vi "filterWheelOpen.vi"   [LabVIEW 2017]
uses:
  globalDevices.vi
  <vilib>/Instr/_visa.llb/VISA Configure Serial Port (Instr).vi
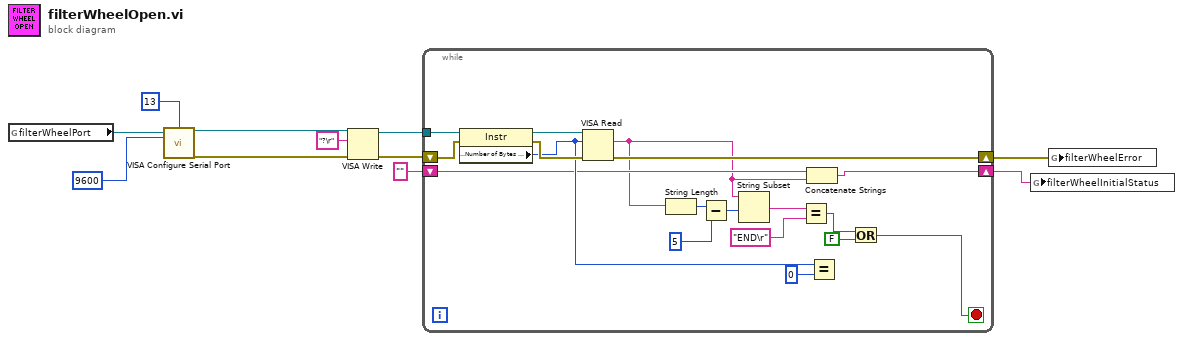
[diagram p0: block diagram]
diagram:
  n1 = global read "globalDevices.vi" "filterWheelPort"() -> (w10:refnum<visa-resource-name>)
  n2 = call-poly "VISA Configure Serial Port"("VISA resource name"=w10, "termination char\n(0xA = '\\n' = LF)"=u8 13 ("termination char\n(0xA = '\\n' = LF)"), "baud rate (9600)"=u32 9600) -> ("VISA resource name out"=w9:refnum<visa-resource-name>, "error out"=w8:errorcluster)  [unwired: 11 in]
  n3 = VISA Write(VISA resource name=w9, write buffer="?\r", error in (no error)=w8) -> (VISA resource name out=w6:refnum<visa-resource-name>, error out=w5:errorcluster)  [unwired: 1 out]
  n4 = while {
    tunnel: w6 -> [w29]
    shift-right: [w15] -> w2
    shift-left: "" -> [w16]
    shift-right: [w14] -> w3
    shift-left: w5 -> [w28]
    stop <- w17 stop-if-true
    n5 = property class="Instr"(reference=w29, error in=w28) -> (reference out=w27:refnum<visa-resource-name>, error out=w26:errorcluster, "Serial Settings:Number of Bytes at Serial Port"=w19:u32)
    n6 = VISA Read(VISA resource name=w27, byte count=w19, error in (no error)=w26) -> (read buffer=w13:string, error out=w14:errorcluster)  [unwired: 2 out]
    n7 = String Length(string=w13) -> (length=w25:i32)
    n8 = Subtract(x=w25, y=5) -> (x-y=w23:i32)
    n9 = String Subset(string=w13, offset (0)=w23) -> (substring=w22:string)  [unwired: 1 in]
    n10 = Equal?(x=w22, y="END\r") -> (x = y?=w20:bool)
    n11 = Concatenate Strings(w16, w13) -> (w15:string)
    n12 = Equal?(x=w19, y=u32 0) -> ()  [unwired: 1 out]
    n13 = Or(x=w20, y=FALSE) -> (x .or. y?=w17:bool)
  }
  n14 = global write "globalDevices.vi" "filterWheelInitialStatus"(w2) -> ()
  n15 = global write "globalDevices.vi" "filterWheelError"(w3) -> ()
